vi "MT Generate QAM Synchronization Parameters (bit array).vi"(0 "QAM system parameters":T1={"samples per symbol (16)"=16, "symbol map"=[]} {"symbol map" format="%.3f"}, 5 "sync bits":i8[](array[numeric]), 11 "error in (no error)":errorcluster, 12 "expected sync location (symbols)":i32=-1, 13 "sync location uncertainty (symbols)":i32=10, 14 "sync indent (symbols)":i32) -> (4 "QAM synchronization parameters":T2 {"sync sequence" format="%.2f"}, 15 "error out":errorcluster)   [LabVIEW 2020, in "niDMT.lvlib"]
doc: "This polymorphic instance generates synchronization parameters for QAM demodulation using a synchronization sequence directly represented by the <B>sync bits</B> array."
uses:
  <vilib>/addons/Modulation/niDMT.lvlib
  <vilib>/addons/Modulation/niAMT.lvlib
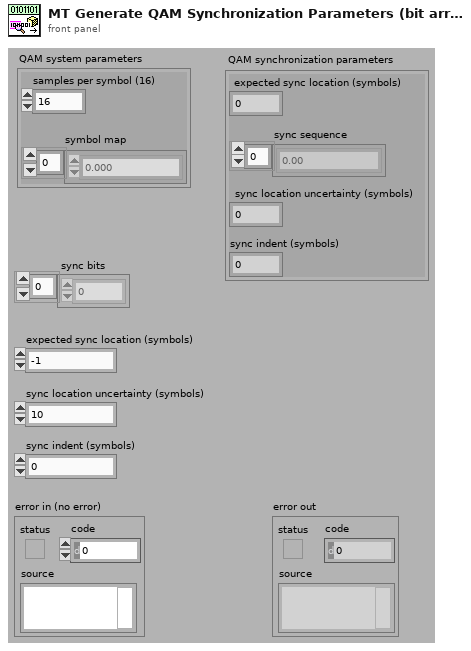
[diagram p1: front panel]
types:
  T1 = cluster{"samples per symbol (16)":i32, "symbol map":cdb[]}
  T2 = cluster{"expected sync location (symbols)":i32, "sync sequence":cdb[], "sync location uncertainty (symbols)":i32, "sync indent (symbols)":i32}
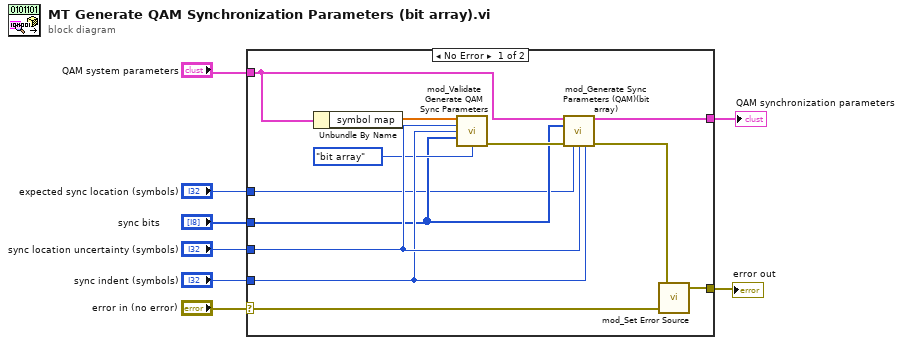
[diagram p0: block diagram]
diagram:
  n1 = case shown="No Error" "error in (no error)" {
    selector: "error in (no error)" -> [w19 w21]
    tunnel: "expected sync location (symbols)" -> [w9 _]
    tunnel: "sync location uncertainty (symbols)" -> [w13 _]
    tunnel: "sync indent (symbols)" -> [w12 _]
    tunnel: "sync bits" -> [w10 _]
    tunnel: [w20 w21] -> w3
    tunnel: "QAM system parameters" -> [w15 _]
    tunnel: [w17 _] -> w1
    frame No Error {
      n2 = Unbundle By Name(w15) -> ("symbol map"=w14:cdb[])
      n3 = call <vilib>:"mod_Validate Generate QAM Sync Parameters.vi"("symbol map"=w14, "sync location uncertainty (symbols)"=w13, "sync indent (symbols)"=w12, "sync bits"=w10, "sync bits specification"=enum16{"bit array", "number array", "number"}."bit array") -> ("error out"=w16:errorcluster)  [unwired: 2 in, 8 out]
      n4 = call <vilib>:"mod_Generate Sync Parameters (QAM)(bit array).vi"("QAM system parameters"=w15, "sync bits"=w10, "error in (no error)"=w16, "expected sync location (symbols)"=w9, "sync location uncertainty (symbols)"=w13, "sync indent (symbols)"=w12) -> ("QAM synchronization parameters"=w17:T2, "error out"=w18:errorcluster)  [unwired: 8 out]
      n5 = call <vilib>:"mod_Set Error Source.vi"("initial error in (no error)"=w19, "final error in (no error)"=w18) -> ("error out"=w20:errorcluster)  [unwired: 3 out]
    }
    frame Error {
    }
  }
  "QAM synchronization parameters" <- w1
  "error out" <- w3
